vi "AcqDataQSMControlModule.vi"() -> ()   [LabVIEW 2013, in "main.lvlib"]
doc: "Læser 4 analoge differentierede datakanaler fra ADC'en og skriver dem til en TDMS-fil. Viser 2 af kanaler i grafer og 2 i søjler."
uses:
  main.lvlib
  Globals/DataAcqRecordPathGlobal.vi
  <vilib>/DAQmx/read.llb/DAQmx Read (Analog 1D DBL NChan 1Samp).vi
  Controls/Enum Globals.ctl
  Controls/Enum Variables.ctl
  Controls/Enum User Events.ctl
  <vilib>/DAQmx/create/channels.llb/DAQmx Create Channel (DO-Digital Output).vi
  <vilib>/DAQmx/write.llb/DAQmx Write (Digital 1D Bool NChan 1Samp 1Line).vi
panel:
  in  "Offset":dbl
  in  "Slide":dbl(slide) min=0.0 max=300.0 step=1.0 scale=0.3..300.0 scale format="%#_3g"
  out "Pressure":dbl(slide) scale=0.0..300.0 scale format="%#.3g"
  out "Red Chart":dbl(graph)
  out "Temperature":dbl caption="Temp"
  out "Blue Chart":dbl(graph)
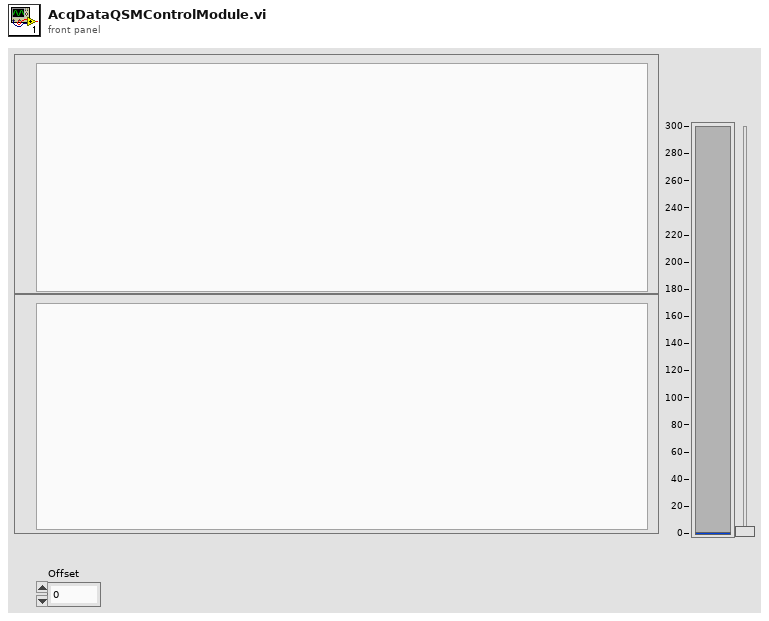
[diagram p1: front panel]
types:
  T1 = typedef "main.lvlib/Enum Globals.ctl" = enum16{"Init", "Set DataPath", "Set Freq", "Get"}
  T2 = typedef "main.lvlib/Enum User Events.ctl" = enum16{"User Event", "Init"}
  T3 = typedef "main.lvlib/Enum Variables.ctl" = enum16{"SetAcqFilter", "GetAcqFilter", "Set Filter", "Get Filter", "Set Height", "Get Height", "Set Blue Pressure", "Get Blue Pressure", "Set Red Pressure", "Get Red Pressure", "Init", "Reset Pressure", "Set Red Cursors", "Get Red Cursors", "Set Blue Cursors", "Get Blue Cursors", "Set Language", "Get Language", "Set Active Graphs", "Get ActiveGraphs", "Set Method", "Get Method", "Set Encryption", "Get Encryption", "Set ExcelVersion", "Get ExcelVersion", "Set DICOM Avail", "Get DICOM Avail", "Set DICOM Encode", "Get DICOM Encode", "Set JournalExport", "Get JournalExport", "Set Sequence", "Get Sequence", "Set DAQ Connected", "Get DAQ Connected", "Set Current Graph", "Get Current Graph", "Set General Settings", "Get Hyphenation", "Set Arm Calc Method", "Get Arm Calc Method", "Set Dicom Tags", "Get Dicom Tags", "Set BT Serial", "Get BT Serial", "Set BT Accepted Serials", "Get BT Accepted Serials", "Get BT License", "Set BT License"}
  T4 = cluster{"Freq Out":i32, "PressureCalibrationFactor":dbl, "RingOut":u16, "data":dbl[], "Value":dbl}
  T5 = cluster{"RingOut":u16, "PressureCalibrationFactor":dbl, "RingOut":u16, "data":dbl[], "Value":dbl}
  T6 = enum16{"open", "open or create", "create or replace", "create", "open (read-only)"}
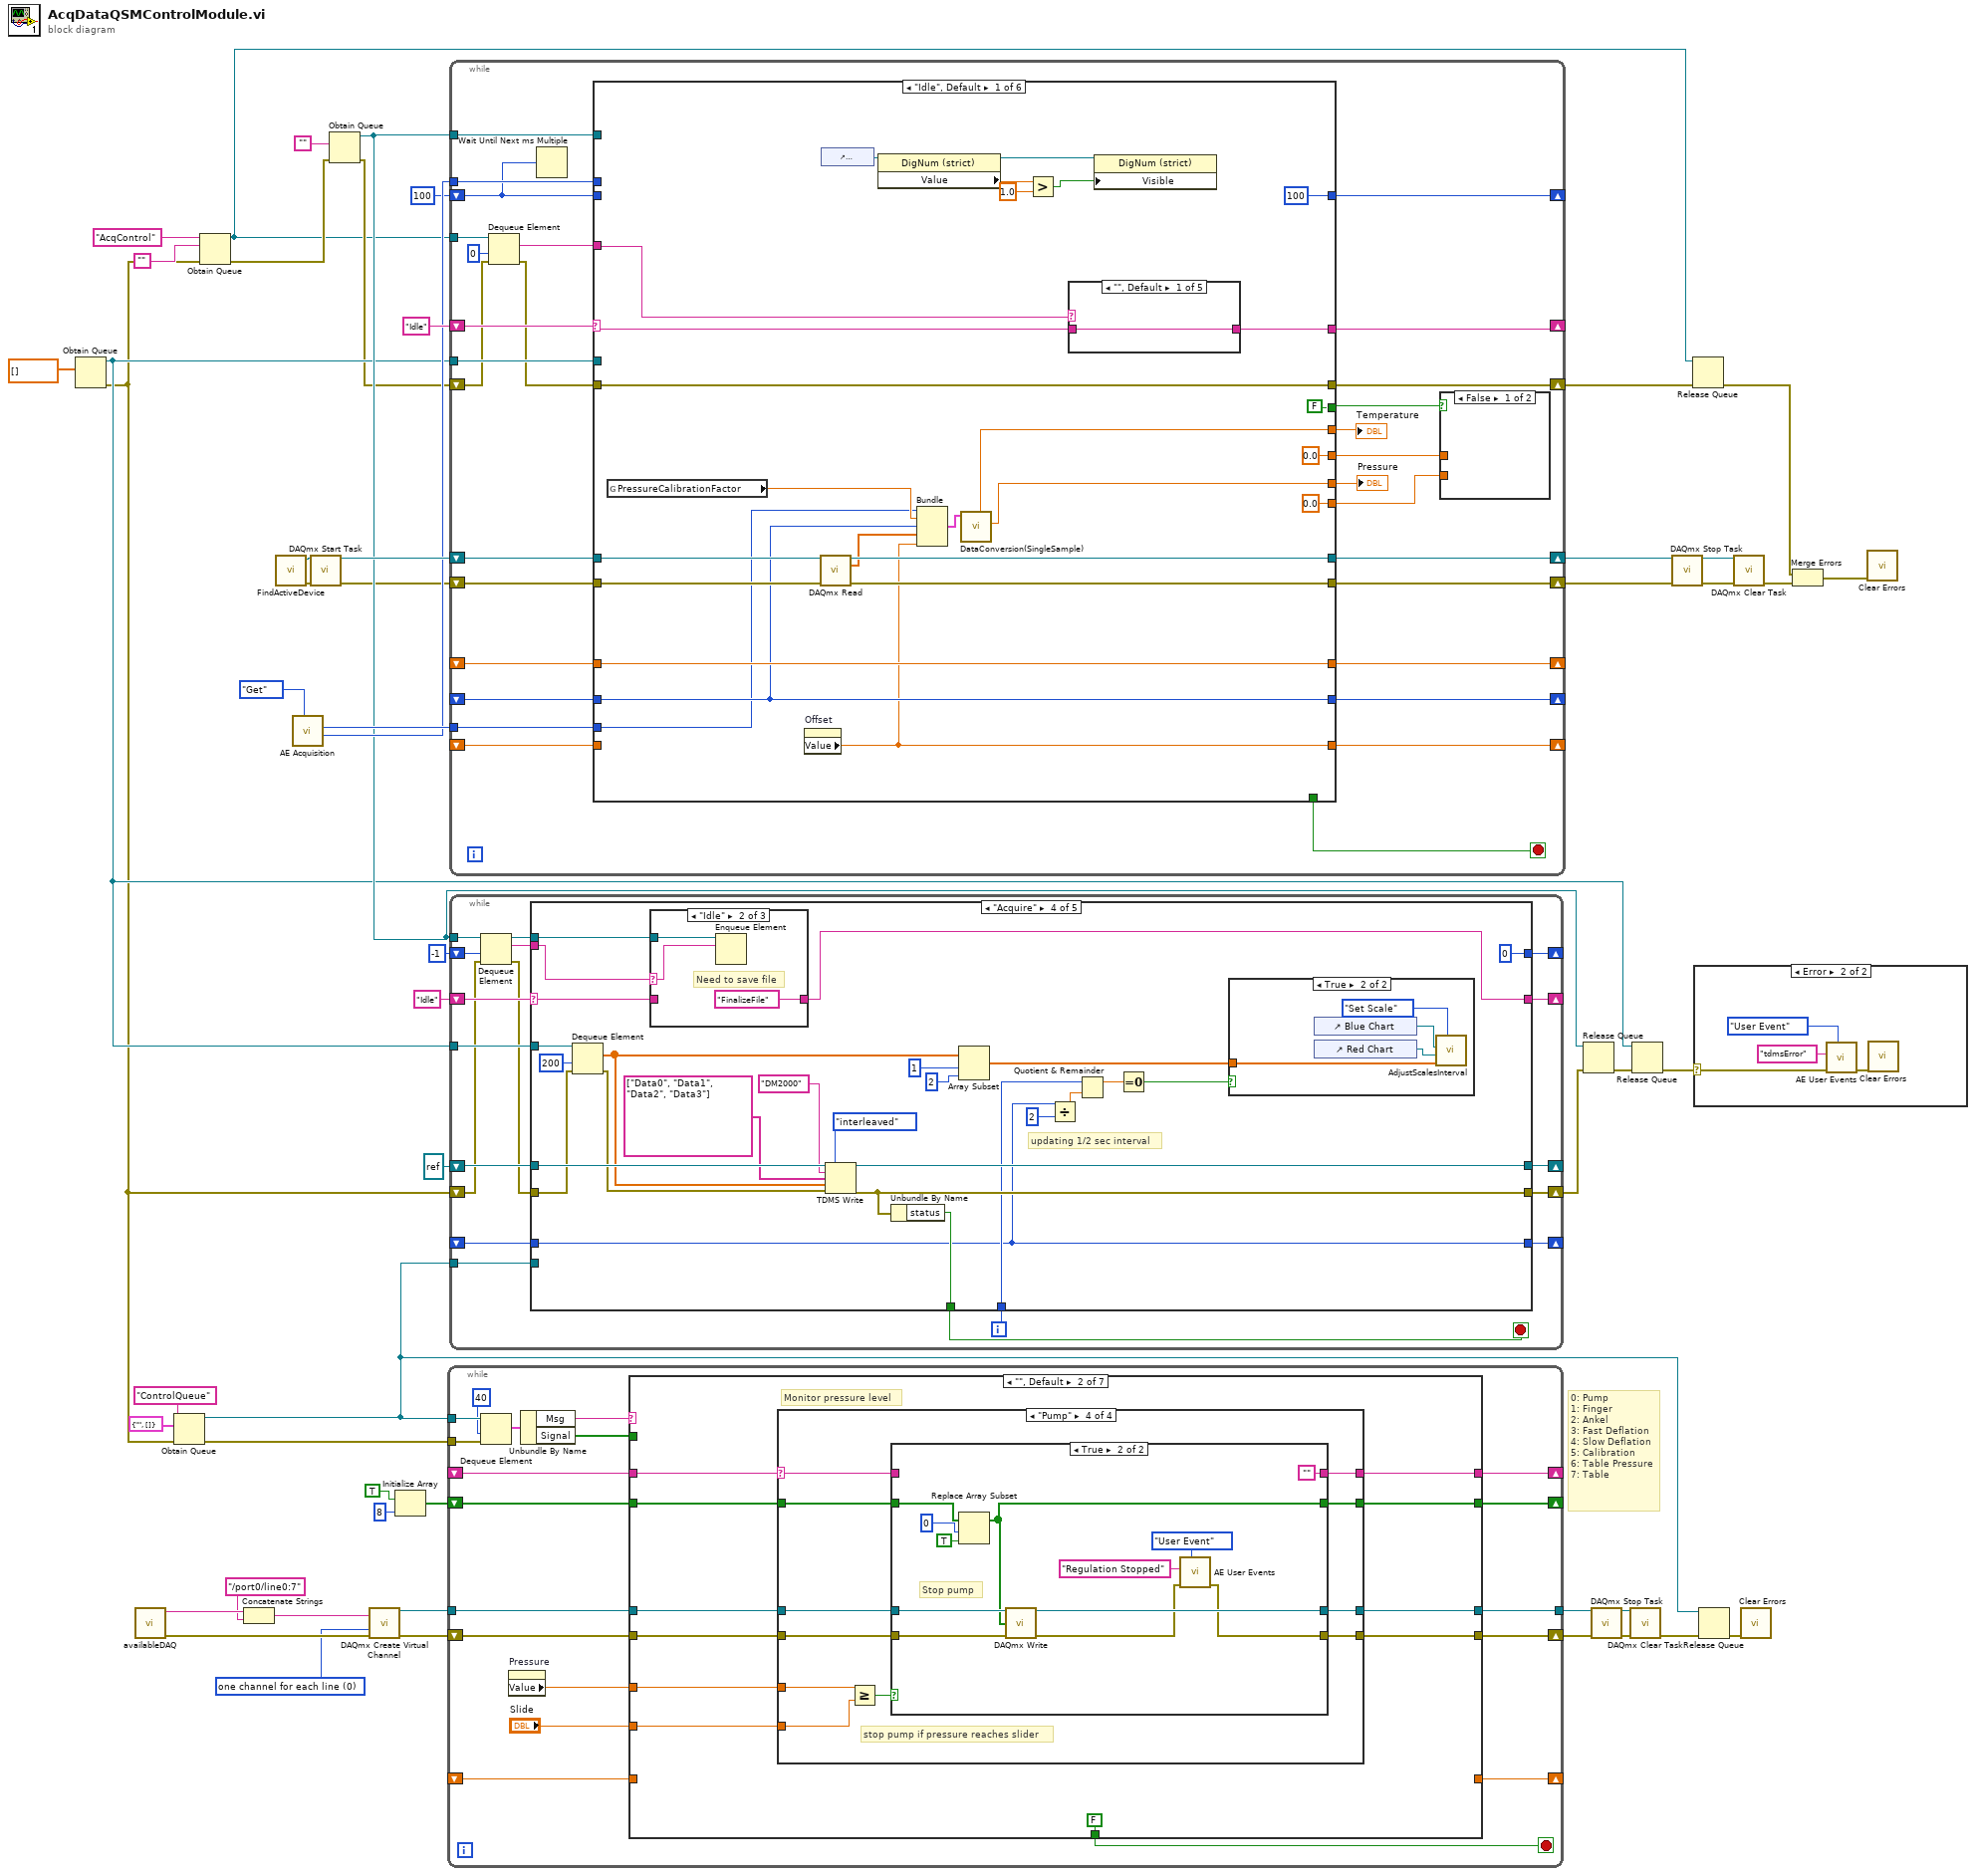
[diagram p0: block diagram]
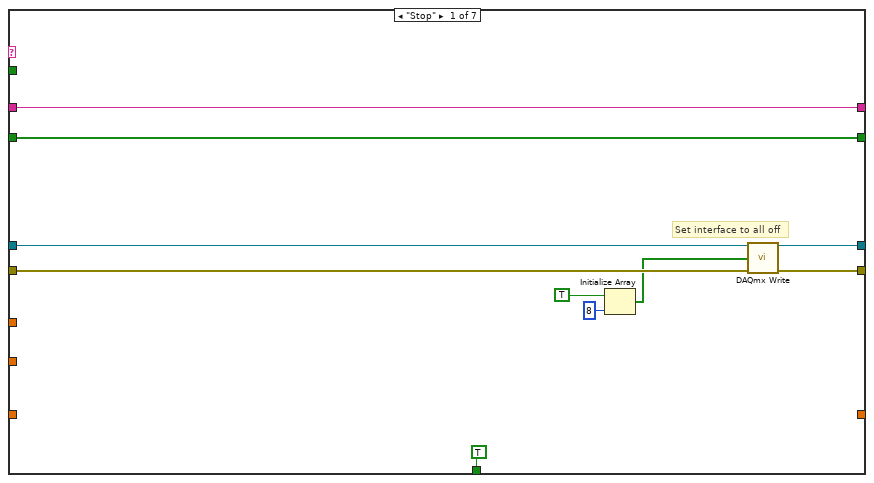
[diagram p2: hidden frame]
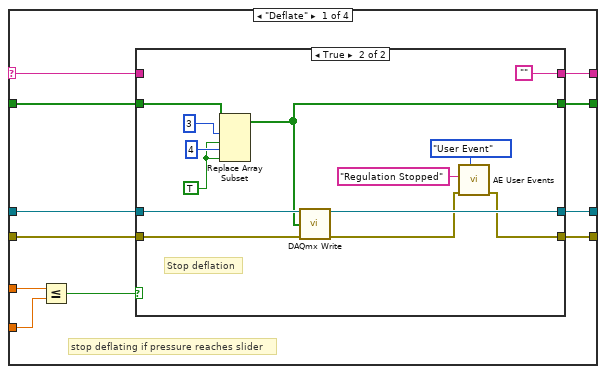
[diagram p3: hidden frame]
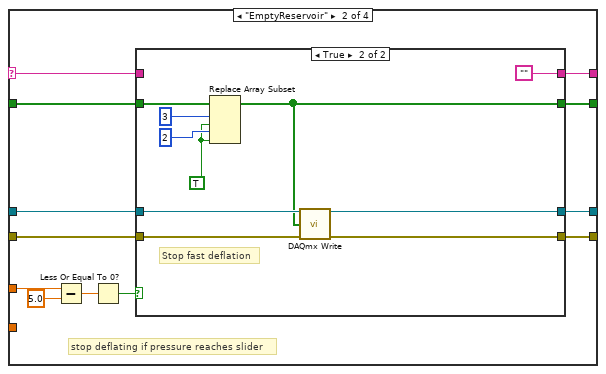
[diagram p5: hidden frame]
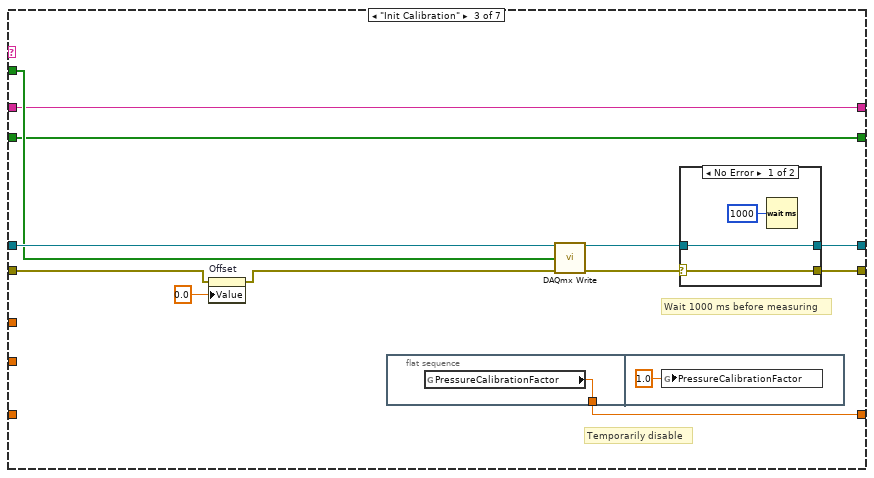
[diagram p9: hidden frame]
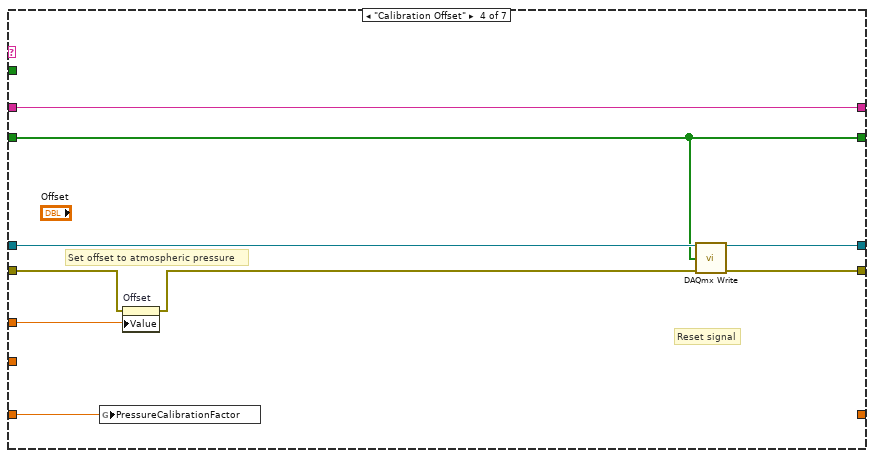
[diagram p11: hidden frame]
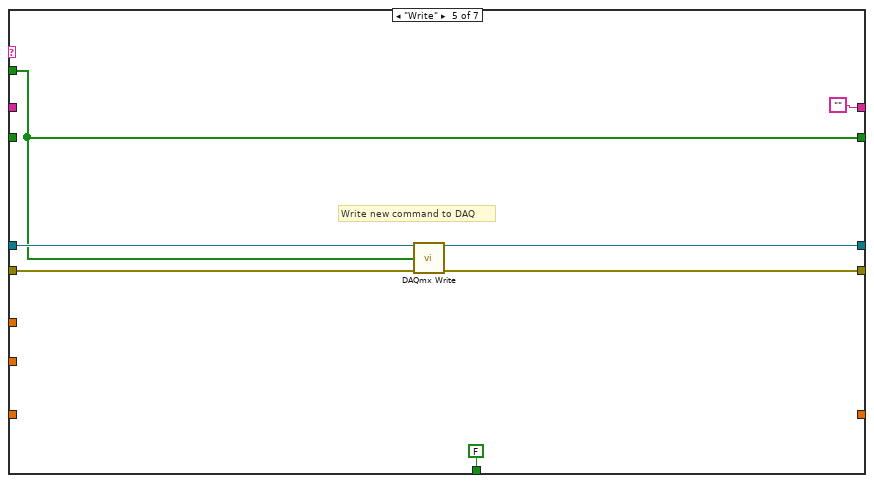
[diagram p12: hidden frame]
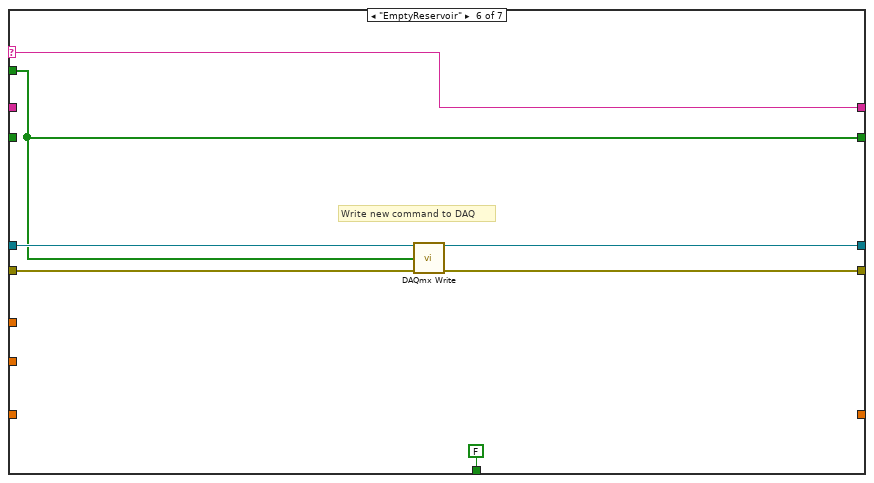
[diagram p13: hidden frame]
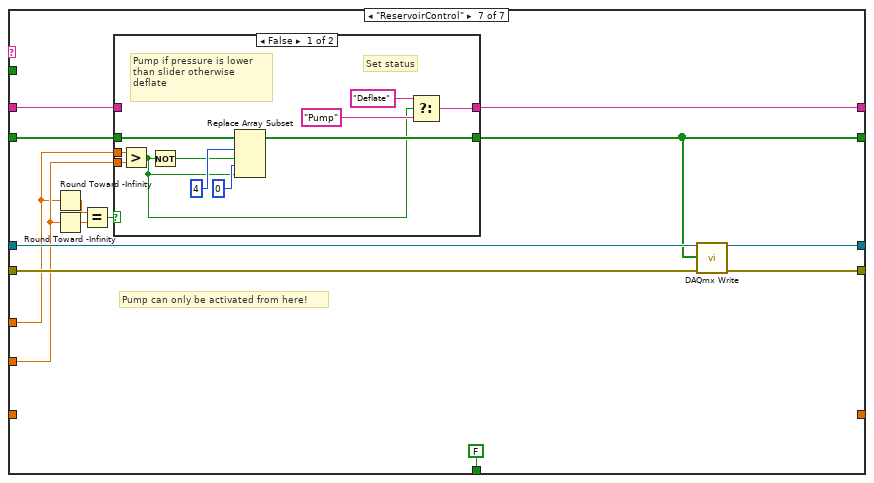
[diagram p14: hidden frame]
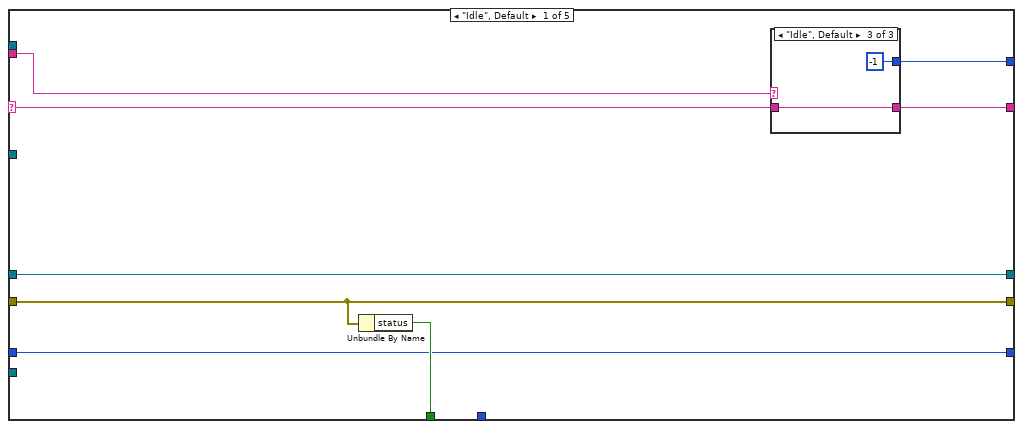
[diagram p17: hidden frame]
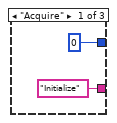
[diagram p18: hidden frame]
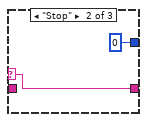
[diagram p19: hidden frame]
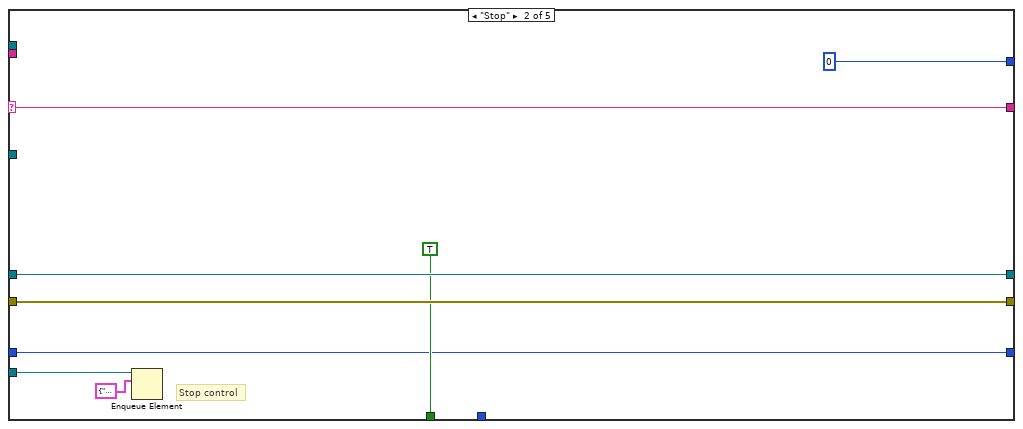
[diagram p20: hidden frame]
diagram:
  w8 = 0 items=["one channel for each line", "one channel for all lines"] ("line grouping")
  # "0: Pump\n1: Finger\n2: Ankel\n3: Fast Deflation\n4: Slow Deflation\n5: Calibration\n6: Table Pressure\n7: Table"
  n1 = Obtain Queue(element data type=dbl[] []) -> (queue out=w34:refnum<queue>, error out=w16:errorcluster)  [unwired: 4 in, 1 out]
  n2 = call "availableDAQ.vi"() -> ("error out"=w19:errorcluster, "DAQmx Device Name"=w21:tag)  [unwired: 10 in]
  n3 = Obtain Queue(name (unnamed)="ControlQueue", element data type=cluster{"Msg":string, "Signal":bool[]} {"Msg"="", "Signal"=[]}, error in (no error)=w16) -> (queue out=w4:refnum<queue>, error out=w7:errorcluster)  [unwired: 2 in, 1 out]
  n4 = Obtain Queue(name (unnamed)="AcqControl", element data type="", error in (no error)=w16) -> (queue out=w29:refnum<queue>, error out=w32:errorcluster)  [unwired: 2 in, 1 out]
  n5 = Concatenate Strings(w21, "/port0/line0:7" ("string")) -> (w18:string)
  n6 = call "FindActiveDevice.vi"() -> ("error out"=w37:errorcluster, "task out"=w38:refnum<k21>)  [unwired: 10 in]
  n7 = call "AE Acquisition.vi"("Action"=Enum_Globals."Get") -> ("Period(ms)"=w42:i32, "Freq Out"=w43:i32)  [unwired: 7 in, 2 out]
  n8 = call <vilib>:"DAQmx Start Task.vi"("task/channels in"=w38, "error in"=w37) -> ("task out"=w49:refnum<k21>, "error out"=w30:errorcluster)  [unwired: 12 in]
  n9 = Obtain Queue(element data type="", error in (no error)=w32) -> (queue out=w35:refnum<queue>, error out=w31:errorcluster)  [unwired: 3 in, 1 out]
  n10 = call-poly <vilib>:"DAQmx Create Virtual Channel.vi"("lines"=w18, "line grouping"=w8, "error in"=w19) -> ("task out"=w15:refnum<k21>, "error out"=w14:errorcluster)  [unwired: 11 in]
  n11 = Initialize Array(TRUE, 8 ("dimension size")) -> (w1:bool[])
  n12 = while {
    tunnel: w4 -> [w72]
    tunnel: w7 -> [w71]
    tunnel: w15 -> [w70]
    shift-right: [w68] -> w12
    shift-left: w14 -> [w69]
    tunnel: [w67] -> w13
    shift-right: [w62] -> _
    shift-left: w1 -> [w61]
    shift-right: [w57] -> _
    shift-left: _ -> [w60]
    shift-right: [w56] -> _
    shift-left: _ -> [w55]
    stop <- w64 stop-if-true
    n13 = Dequeue Element(queue=w72, timeout in ms (-1)=40, error in (no error)=w71) -> (element=w66:cluster{"Msg":string, "Signal":bool[]})  [unwired: 3 out]
    n14 = property on="Pressure" class="Slide (strict)"() -> ("Value"=w59:dbl)  [unwired: 2 in, 2 out]
    n15 = Unbundle By Name(w66) -> ("Msg"=w65:string, "Signal"=w54:bool[])
    n16 = case shown="\"\", Default" w65 {
      selector: w65 -> [_ _ _ _ _ w214 _]
      tunnel: w70 -> [w78 w92 w190 w203 w213 w220 w234]
      tunnel: w69 -> [w77 w91 w182 w200 w212 w219 w233]
      tunnel: [w79 w89 w185 w204 w210 w217 w231] -> w68
      tunnel: [w80 w90 w183 w205 w211 w218 w232] -> w67
      tunnel: [TRUE FALSE _ _ FALSE FALSE FALSE] -> w64
      tunnel: w54 -> [_ _ w189 _ w208 w215 _]
      tunnel: [w81 w87 w187 w202 w208 w215 w223] -> w62
      tunnel: w61 -> [w81 w88 w187 w202 _ _ w224]
      tunnel: w60 -> [w73 w86 w188 w206 _ _ w221]
      tunnel: w59 -> [_ w85 _ w201 _ _ w225]
      tunnel: "Slide" -> [_ w84 _ _ _ _ w227]
      tunnel: [w73 w83 w188 w206 "" w214 w222] -> w57
      tunnel: [_ _ w179 _ _ _ _] -> w56
      tunnel: w55 -> [_ _ _ w198 _ _ _]
      frame "Stop" {
        # "Set interface to all off"
        n17 = Initialize Array(TRUE, 8 ("dimension size")) -> (w74:bool[])
        n18 = call-poly <vilib>:"DAQmx Write.vi"("task/channels in"=w78, "data"=w74, "error in"=w77) -> ("task out"=w80:refnum<k21>, "error out"=w79:errorcluster)  [unwired: 10 in, 1 out]
      }
      frame "", Default {
        # "Monitor pressure level"
        n19 = case shown="\"Pump\"" w86 {
          selector: w86 -> [w95 w126 w151 w153]
          tunnel: w92 -> [w99 w128 w149 w162]
          tunnel: w91 -> [w100 w129 w148 w161]
          tunnel: [w102 w131 w149 w160] -> w90
          tunnel: [w101 w130 w148 w159] -> w89
          tunnel: w88 -> [w104 w133 w150 w157]
          tunnel: [w103 w132 w150 w156] -> w87
          tunnel: [w96 w127 w151 w152] -> w83
          tunnel: w85 -> [w97 w124 _ w155]
          tunnel: w84 -> [w98 _ _ w154]
          frame "Deflate" {
            # "stop deflating if pressure reaches slider"
            n20 = Less Or Equal?(x=w97, y=w98) -> (x <= y?=w94:bool)
            n21 = case shown="True" w94 {
              tunnel: w99 -> [w108 w121]
              tunnel: w100 -> [w107 w120]
              tunnel: [w108 w119] -> w102
              tunnel: [w107 w112] -> w101
              tunnel: w104 -> [w106 w118]
              tunnel: [w106 w109] -> w103
              tunnel: [w105 ""] -> w96
              tunnel: w95 -> [w105 _]
              frame False {
              }
              frame True {
                w110 = TRUE ("new element/subarray")
                # "Stop deflation"
                n22 = Replace Array Subset(array=w118, new element #1=w110, index #1=3 ("index"), new element #2=w110, index #2=4) -> (w109:bool[])
                n23 = call-poly <vilib>:"DAQmx Write.vi"("task/channels in"=w121, "data"=w109, "error in"=w120) -> ("task out"=w119:refnum<k21>, "error out"=w113:errorcluster)  [unwired: 10 in, 1 out]
                n24 = call "AE User Events.vi"("Action"=Enum_User_Events."User Event", "error in (no error)"=w113, "User Event"="Regulation Stopped") -> ("error out"=w112:errorcluster)  [unwired: 7 in, 1 out]
              }
            }
          }
          frame "EmptyReservoir" {
            # "stop deflating if pressure reaches slider"
            n25 = Subtract(x=w124, y=5.0) -> (x-y=w123:dbl)
            n26 = Less Or Equal To 0?(x=w123) -> (x <= 0?=w125:bool)
            n27 = case shown="True" w125 {
              tunnel: w128 -> [w137 w147]
              tunnel: w129 -> [w136 w146]
              tunnel: [w137 w145] -> w131
              tunnel: [w136 w141] -> w130
              tunnel: w133 -> [w135 w144]
              tunnel: [w135 w138] -> w132
              tunnel: [w134 ""] -> w127
              tunnel: w126 -> [w134 _]
              frame False {
              }
              frame True {
                w139 = TRUE ("new element/subarray")
                # "Stop fast deflation"
                n28 = Replace Array Subset(array=w144, new element #1=w139, index #1=3 ("index"), new element #2=w139, index #2=2 ("index")) -> (w138:bool[])
                n29 = call-poly <vilib>:"DAQmx Write.vi"("task/channels in"=w147, "data"=w138, "error in"=w146) -> ("task out"=w145:refnum<k21>, "error out"=w141:errorcluster)  [unwired: 10 in, 1 out]
              }
            }
          }
          frame "", Default {
          }
          frame "Pump" {
            # "stop pump if pressure reaches slider"
            n30 = Greater Or Equal?(x=w155, y=w154) -> (x >= y?=w158:bool)
            n31 = case shown="True" w158 {
              tunnel: w162 -> [w166 w178]
              tunnel: w161 -> [w165 w177]
              tunnel: [w166 w176] -> w160
              tunnel: [w165 w170] -> w159
              tunnel: w157 -> [w164 w173]
              tunnel: [w164 w167] -> w156
              tunnel: w153 -> [w163 _]
              tunnel: [w163 ""] -> w152
              frame False {
              }
              frame True {
                # "Stop pump"
                n32 = Replace Array Subset(array=w173, new element=TRUE ("new element/subarray"), index=0) -> (w167:bool[])
                n33 = call-poly <vilib>:"DAQmx Write.vi"("task/channels in"=w178, "data"=w167, "error in"=w177) -> ("task out"=w176:refnum<k21>, "error out"=w171:errorcluster)  [unwired: 10 in, 1 out]
                n34 = call "AE User Events.vi"("Action"=Enum_User_Events."User Event", "error in (no error)"=w171, "User Event"="Regulation Stopped") -> ("error out"=w170:errorcluster)  [unwired: 7 in, 1 out]
              }
            }
          }
        }
      }
      frame "Init Calibration" {
        # "Temporarily disable"
        # "Wait 1000 ms before measuring"
        n35 = property on="Offset" class="DigNum (strict)"(error in=w182, "Value"=0.0 ("Offset")) -> (error out=w181:errorcluster)  [unwired: 1 in, 1 out]
        n36 = flat-sequence {
          tunnel: [w191] -> w179
          frame #0 {
            n37 = global read "DataAcqRecordPathGlobal.vi" "PressureCalibrationFactor"() -> (w191:dbl)
          }
          frame #1 {
            n38 = global write "DataAcqRecordPathGlobal.vi" "PressureCalibrationFactor"(1.0 ("PressureCalibrationFactor")) -> ()
          }
        }
        n39 = call-poly <vilib>:"DAQmx Write.vi"("task/channels in"=w190, "data"=w189, "error in"=w181) -> ("task out"=w184:refnum<k21>, "error out"=w186:errorcluster)  [unwired: 10 in, 1 out]
        n40 = case shown="No Error" w186 {
          selector: w186 -> [w195 w197]
          tunnel: [w195 w197] -> w185
          tunnel: [w194 w196] -> w183
          tunnel: w184 -> [w194 w196]
          frame No Error {
            n41 = Wait (ms)(milliseconds to wait=u32 1000) -> ()  [unwired: 1 out]
          }
          frame Error {
          }
        }
      }
      frame "Calibration Offset" {
        # "Reset signal"
        # "Set offset to atmospheric pressure"
        n42 = global write "DataAcqRecordPathGlobal.vi" "PressureCalibrationFactor"(w198) -> ()
        n43 = property on="Offset" class="DigNum (strict)"(error in=w200, "Value"=w201) -> (error out=w199:errorcluster)  [unwired: 1 in, 1 out]
        n44 = call-poly <vilib>:"DAQmx Write.vi"("task/channels in"=w203, "data"=w202, "error in"=w199) -> ("task out"=w205:refnum<k21>, "error out"=w204:errorcluster)  [unwired: 10 in, 1 out]
      }
      frame "Write" {
        # "Write new command to DAQ"
        n45 = call-poly <vilib>:"DAQmx Write.vi"("task/channels in"=w213, "data"=w208, "error in"=w212) -> ("task out"=w211:refnum<k21>, "error out"=w210:errorcluster)  [unwired: 10 in, 1 out]
      }
      frame "EmptyReservoir" {
        # "Write new command to DAQ"
        n46 = call-poly <vilib>:"DAQmx Write.vi"("task/channels in"=w220, "data"=w215, "error in"=w219) -> ("task out"=w218:refnum<k21>, "error out"=w217:errorcluster)  [unwired: 10 in, 1 out]
      }
      frame "ReservoirControl" {
        # "Pump can only be activated from here!"
        n47 = Round Toward -Infinity(1:w225) -> (0:w226:dbl)
        n48 = Round Toward -Infinity(1:w227) -> (0:w228:dbl)
        n49 = Equal?(x=w226, y=w228) -> (x = y?=w229:bool)
        n50 = case shown="False" w229 {
          tunnel: w224 -> [w245 w247]
          tunnel: w225 -> [w243 _]
          tunnel: w227 -> [w242 _]
          tunnel: [w238 w247] -> w223
          tunnel: [w239 w246] -> w222
          tunnel: w221 -> [_ w246]
          frame False {
            # "Set status"
            # "Pump if pressure is lower than slider otherwise deflate"
            n51 = Greater?(x=w243, y=w242) -> (0:w236:bool)
            n52 = Not(x=w236) -> (.not. x?=w240:bool)
            n53 = Replace Array Subset(array=w245, new element #1=w240, index #1=4 ("index"), new element #2=w236, index #2=0 ("index")) -> (w238:bool[])
            n54 = Select(t="Deflate", s=w236, f="Pump") -> (s? t:f=w239:string)
          }
          frame True {
            # "Ignore if pressure = slide"
          }
        }
        n55 = call-poly <vilib>:"DAQmx Write.vi"("task/channels in"=w234, "data"=w223, "error in"=w233) -> ("task out"=w232:refnum<k21>, "error out"=w231:errorcluster)  [unwired: 10 in, 1 out]
      }
    }
  }
  n56 = while {
    shift-right: [w253] -> w50
    shift-left: w49 -> [w277]
    shift-right: [w252] -> w53
    shift-left: w30 -> [w276]
    shift-right: [w270] -> _
    shift-left: 100 ("Period(ms)") -> [w251]
    shift-right: [w255] -> w28
    shift-left: w31 -> [w257]
    shift-right: [w273] -> _
    shift-left: "Idle" -> [w274]
    tunnel: w43 -> [w269]
    tunnel: w42 -> [w268]
    shift-right: [w267] -> _
    shift-left: _ -> [w266]
    shift-right: [w262] -> _
    shift-left: _ -> [w261]
    tunnel: w29 -> [w260]
    tunnel: w35 -> [w258]
    tunnel: w34 -> [w275]
    shift-right: [w248] -> _
    shift-left: _ -> [w249]
    stop <- w254 stop-if-true
    n57 = Dequeue Element(queue=w260, timeout in ms (-1)=0, error in (no error)=w257) -> (element=w259:string, error out=w256:errorcluster)  [unwired: 2 out]
    n58 = Wait Until Next ms Multiple(millisecond multiple=w251) -> ()  [unwired: 1 out]
    n59 = case shown="\"Idle\", Default" w274 {
      selector: w274 -> [w298 _ w358 _ w410 w431]
      tunnel: [w305 w326 w366 w380 w416 w429] -> w252
      tunnel: w277 -> [w304 w329 w365 w383 w415 w430]
      tunnel: [w303 w330 w364 w384 w414 w430] -> w253
      tunnel: w276 -> [w302 w331 w363 w385 w413 w429]
      tunnel: [_ _ _ _ _ TRUE ("status")] -> w254
      tunnel: [100 w320 w357 w377 w404 w428] -> w270
      tunnel: w251 -> [_ _ w357 _ w404 w428]
      tunnel: w275 -> [_ _ w361 _ _ _]
      tunnel: [w301 w317 w348 w396 w409 w421] -> w255
      tunnel: w256 -> [w301 w317 w362 w396 w409 w421]
      tunnel: [w286 0.0 w353 0.0 w406 _] -> w272
      tunnel: [w300 0.0 ("Temperature") w360 0.0 ("Temperature") w412 _] -> w271
      tunnel: [w297 "Acquire" w359 "Test" w411 w431] -> w273
      tunnel: [0.0 ("Blue Data") _ w355 _ w407 _] -> w263
      tunnel: [0.0 ("Red Data") _ w354 _ w408 _] -> w264
      tunnel: [FALSE FALSE TRUE FALSE TRUE FALSE] -> w265
      tunnel: w269 -> [w281 w324 w344 w375 w399 _]
      tunnel: w268 -> [_ w320 _ w377 _ _]
      tunnel: [w288 w314 w345 w374 w398 w425] -> w267
      tunnel: w266 -> [w288 _ w345 _ w398 w425]
      tunnel: [w283 w313 w346 w372 w397 w424] -> w262
      tunnel: w261 -> [w283 w315 w346 _ w397 w424]
      tunnel: w259 -> [w287 _ w350 _ w403 _]
      tunnel: w258 -> [_ w319 w349 _ _ w423]
      tunnel: w249 -> [_ w311 w342 w371 w400 w420]
      tunnel: [w280 w311 w342 w371 w400 w420] -> w248
      frame "Idle", Default {
        n60 = global read "DataAcqRecordPathGlobal.vi" "PressureCalibrationFactor"() -> (w282:dbl)
        n61 = property on="Offset" class="DigNum (strict)"() -> ("Value"=w280:dbl)  [unwired: 2 in, 2 out]
        n62 = call-poly <vilib>:"DAQmx Read.vi"("task/channels in"=w304, "error in"=w302) -> ("task out"=w303:refnum<k21>, "data"=w284:dbl[], "error out"=w305:errorcluster)  [unwired: 11 in]
        n63 = control-ref of="Temperature"() -> (w293:refnum<vi>)
        n64 = property class="DigNum (strict)"(reference=w293) -> (reference out=w292:refnum<vi>, "Value"=w291:dbl)  [unwired: 1 in, 1 out]
        n65 = Bundle("Freq Out"=w281, "PressureCalibrationFactor"=w282, "RingOut"=w283, "data"=w284, "Value"=w280) -> (w285:T4)  [unwired: 1 in]
        n66 = call "DataConversion(SingleSample).vi"("input cluster"=w285) -> ("Temperature"=w300:dbl, "Pressure"=w286:dbl)  [unwired: 5 in, 3 out]
        n67 = Greater?(x=w291, y=1.0) -> (0:w289:bool)
        n68 = case shown="\"\", Default" w287 {
          tunnel: w298 -> [w306 w307 _ _ _]
          tunnel: [w306 w307 "Initialize" "Stop" "InitTest"] -> w297
          frame "", Default {
          }
          frame "Idle" {
          }
          frame "Acquire" {
          }
          frame "Stop" {
          }
          frame "Test" {
          }
        }
        n69 = property class="DigNum (strict)"(reference=w292, "Visible"=w289) -> ()  [unwired: 1 in, 2 out]
      }
      frame "Initialize" {
        w337 = dbl[] [] ("Value")
        n70 = global read "DataAcqRecordPathGlobal.vi" "PressureCalibrationFactor"() -> (w314:dbl)
        n71 = Enqueue Element(queue=w319, element="Acquire") -> ()  [unwired: 2 in, 3 out]
        n72 = Reciprocal(x=w324) -> (1/x=w336:dbl)
        n73 = control-ref of="Red Chart"() -> (w328:refnum<vi>)
        n74 = control-ref of="Blue Chart"() -> (w327:refnum<vi>)
        n75 = call "AE Variables.vi"("Action"=Enum_Variables."Get ActiveGraphs") -> ("RingOut"=w313:u16)  [unwired: 11 in, 7 out]
        n76 = call-poly <vilib>:"DAQmx Read.vi"("task/channels in"=w329, "error in"=w331) -> ("task out"=w330:refnum<k21>, "data"=w312:dbl[], "error out"=w326:errorcluster)  [unwired: 11 in]
        n77 = property class="WFChart (strict)"(reference=w328, "History Data"=w337, "XScale.Multiplier"=w336) -> (reference out=w323:refnum<vi>)  [unwired: 1 in, 1 out]
        n78 = property class="WFChart (strict)"(reference=w327, "History Data"=w337, "XScale.Multiplier"=w336) -> (reference out=w322:refnum<vi>)  [unwired: 1 in, 1 out]
        n79 = Bundle("RingOut"=w315, "PressureCalibrationFactor"=w314, "RingOut"=w313, "data"=w312, "Value"=w311) -> (w316:T5)  [unwired: 1 in]
        n80 = call "DataConversion(SingleSample).vi"("input cluster"=w316, "Init"=TRUE) -> ("Red Data"=w333:dbl, "Blue Data"=w334:dbl)  [unwired: 4 in, 3 out]
        n81 = Build Array(w334, w333) -> (w332:dbl[])
        n82 = call "AdjustScalesInterval.vi"("Action"=enum16{"Init", "Set Scale"}."Init", "Data"=w332, "WFChart Refnum 2"=w323, "WFChart Refnum"=w322) -> ()  [unwired: 8 in]
      }
      frame "Acquire" {
        n83 = call-poly <vilib>:"DAQmx Read.vi"("task/channels in"=w365, "error in"=w363) -> ("task out"=w364:refnum<k21>, "data"=w347:dbl[], "error out"=w366:errorcluster)  [unwired: 11 in]
        n84 = Bundle("Freq Out"=w344, "PressureCalibrationFactor"=w345, "RingOut"=w346, "data"=w347, "Value"=w342) -> (w343:T4)  [unwired: 1 in]
        n85 = call "DataConversion(SingleSample).vi"("input cluster"=w343, "Init"=FALSE) -> ("Temperature"=w360:dbl, "All Data"=w356:dbl[], "Red Data"=w354:dbl, "Pressure"=w353:dbl, "Blue Data"=w355:dbl)  [unwired: 4 in]
        n86 = Enqueue Element(queue=w361, element=w356, error in (no error)=w362) -> (error out=w348:errorcluster)  [unwired: 1 in, 2 out]
        n87 = case shown="\"\", Default" w350 {
          selector: w350 -> [_ w368 w370]
          tunnel: [w367 w368 w370] -> w359
          tunnel: w358 -> [w367 _ _]
          tunnel: w349 -> [_ w369 _]
          frame "", Default {
          }
          frame "Idle" {
            n88 = Enqueue Element(queue=w369, element=w368) -> ()  [unwired: 2 in, 3 out]
          }
          frame "Stop" {
          }
        }
      }
      frame "InitTest" {
        w391 = dbl[] [] ("Value")
        n89 = Reciprocal(x=w375) -> (1/x=w390:dbl)
        n90 = global read "DataAcqRecordPathGlobal.vi" "PressureCalibrationFactor"() -> (w374:dbl)
        n91 = call "AE Variables.vi"("Action"=Enum_Variables."Get ActiveGraphs") -> ("RingOut"=w372:u16)  [unwired: 11 in, 7 out]
        n92 = control-ref of="Red Chart"() -> (w382:refnum<vi>)
        n93 = control-ref of="Blue Chart"() -> (w381:refnum<vi>)
        n94 = call-poly <vilib>:"DAQmx Read.vi"("task/channels in"=w383, "error in"=w385) -> ("task out"=w384:refnum<k21>, "data"=w373:dbl[], "error out"=w380:errorcluster)  [unwired: 11 in]
        n95 = Bundle("Freq Out"=w375, "PressureCalibrationFactor"=w374, "RingOut"=w372, "data"=w373, "Value"=w371) -> (w376:T4)  [unwired: 1 in]
        n96 = call "DataConversion(SingleSample).vi"("input cluster"=w376, "Init"=TRUE) -> ("Red Data"=w387:dbl, "Blue Data"=w388:dbl)  [unwired: 4 in, 3 out]
        n97 = Build Array(w388, w387) -> (w386:dbl[])
        n98 = property class="WFChart (strict)"(reference=w382, "History Data"=w391, "XScale.Multiplier"=w390) -> ()  [unwired: 1 in, 2 out]
        n99 = property class="WFChart (strict)"(reference=w381, "History Data"=w391, "XScale.Multiplier"=w390) -> ()  [unwired: 1 in, 2 out]
        n100 = call "AdjustScalesInterval.vi"("Action"=enum16{"Init", "Set Scale"}."Init", "Data"=w386, "WFChart Refnum 2"=w382, "WFChart Refnum"=w381) -> ()  [unwired: 8 in]
      }
      frame "Test" {
        n101 = call-poly <vilib>:"DAQmx Read.vi"("task/channels in"=w415, "error in"=w413) -> ("task out"=w414:refnum<k21>, "data"=w401:dbl[], "error out"=w416:errorcluster)  [unwired: 11 in]
        n102 = Bundle("Freq Out"=w399, "PressureCalibrationFactor"=w398, "RingOut"=w397, "data"=w401, "Value"=w400) -> (w402:T4)  [unwired: 1 in]
        n103 = call "DataConversion(SingleSample).vi"("input cluster"=w402) -> ("Temperature"=w412:dbl, "Red Data"=w408:dbl, "Pressure"=w406:dbl, "Blue Data"=w407:dbl)  [unwired: 5 in, 1 out]
        n104 = case shown="\"False\", Default" w403 {
          tunnel: [w417 "Idle" "Stop"] -> w411
          tunnel: w410 -> [w417 _ _]
          frame "False", Default {
          }
          frame "Idle" {
          }
          frame "Stop" {
          }
        }
      }
      frame "Stop" {
        n105 = Enqueue Element(queue=w423, element="Stop") -> ()  [unwired: 2 in, 3 out]
      }
    }
    "Pressure" <- w272
    "Temperature" <- w271
    n106 = case shown="False" w265 {
      tunnel: w264 -> [_ w279]
      tunnel: w263 -> [_ w278]
      frame False {
      }
      frame True {
        "Blue Chart" <- w278
        "Red Chart" <- w279
      }
    }
  }
  n107 = while {
    tunnel: w34 -> [w449]
    shift-right: [w447] -> _
    shift-left: refnum<k34> refnum ("tdms file out") -> [w448]
    shift-right: [w446] -> w45
    shift-left: w16 -> [w435]
    shift-right: [w443] -> _
    shift-left: "Idle" -> [w444]
    shift-right: [w441] -> _
    shift-left: _ -> [w440]
    tunnel: w35 -> [w439]
    shift-right: [w436] -> _
    shift-left: -1 -> [w437]
    tunnel: w4 -> [w432]
    i -> [w442]
    stop <- w445 stop-if-true
    n108 = Dequeue Element(queue=w439, timeout in ms (-1)=w437, error in (no error)=w435) -> (queue out=w433:refnum<queue>, element=w438:string, error out=w434:errorcluster)  [unwired: 1 out]
    n109 = case shown="\"Acquire\"" w444 {
      selector: w444 -> [w455 w471 _ w502 _]
      tunnel: w449 -> [_ _ _ w503 w521]
      tunnel: w448 -> [w457 w470 _ w506 w525]
      tunnel: [w457 w470 w476 w507 w525] -> w447
      tunnel: [w454 w469 w477 w505 w526] -> w446
      tunnel: w434 -> [w454 w469 w479 w499 w520]
      tunnel: [w453 TRUE ("status") w478 w504 w527] -> w445
      tunnel: [w456 w471 "Acquire" w496 w522] -> w443
      tunnel: w442 -> [_ _ _ w491 _]
      tunnel: [w452 w467 w473 w486 w524] -> w441
      tunnel: w440 -> [w452 w467 _ w486 w524]
      tunnel: w438 -> [w451 _ _ w484 w522]
      tunnel: [w450 0 0 0 100] -> w436
      tunnel: w433 -> [_ _ _ w483 _]
      tunnel: w432 -> [_ w465 _ _ _]
      frame "Idle", Default {
        n110 = Unbundle By Name(w454) -> ("status"=w453:bool)
        n111 = case shown="\"Idle\", Default" w451 {
          selector: w451 -> [_ w460 _]
          tunnel: ["Initialize" w460 w463] -> w456
          tunnel: w455 -> [_ _ w463]
          tunnel: [0 0 -1] -> w450
          frame "Acquire" {
          }
          frame "Stop" {
          }
          frame "Idle", Default {
          }
        }
      }
      frame "Stop" {
        # "Stop control"
        n112 = Enqueue Element(queue=w465, element=cluster{"Msg":string, "Signal":bool[]} {"Msg"="Stop", "Signal"=[]}) -> ()  [unwired: 2 in, 3 out]
      }
      frame "Initialize" {
        n113 = global read "DataAcqRecordPathGlobal.vi" "DataAcqRecordPath"() -> (w481:path)
        n114 = TDMS Open(8:w479, 10:T6."create or replace" ("operation (0:open)"), 11:w481) -> (0:w477:errorcluster, 3:w476:refnum<k34>)  [unwired: 4 in]
        n115 = Unbundle By Name(w477) -> ("status"=w478:bool)
        n116 = call "AE Acquisition.vi"("Action"=Enum_Globals."Get") -> ("Freq Out"=w473:i32)  [unwired: 7 in, 3 out]
      }
      frame "Acquire" {
        # "updating 1/2 sec interval"
        n117 = Dequeue Element(queue=w503, timeout in ms (-1)=200, error in (no error)=w499) -> (element=w490:dbl[], error out=w498:errorcluster)  [unwired: 2 out]
        n118 = case shown="\"Idle\"" w484 {
          selector: w484 -> [_ w513 w516]
          tunnel: [w512 "FinalizeFile" "FinalizeFile"] -> w496
          tunnel: w502 -> [w512 _ _]
          tunnel: w483 -> [_ w514 w517]
          frame "", Default {
          }
          frame "Idle" {
            # "Need to save file"
            n119 = Enqueue Element(queue=w514, element=w513) -> ()  [unwired: 2 in, 3 out]
          }
          frame "Stop" {
            # "Need to save file"
            n120 = Enqueue Element(queue=w517, element=w516) -> ()  [unwired: 2 in, 3 out]
          }
        }
        n121 = TDMS Write(0:w506, 1:enum16{"decimated", "interleaved"}."interleaved" ("data layout (0:decimated)"), 5:"DM2000", 7:string[] ["Data0", "Data1", "Data2", "Data3"], 9:w490, 11:w498) -> (4:w507:refnum<k34>, 15:w505:errorcluster)  [unwired: 2 out]
        n122 = Unbundle By Name(w505) -> ("status"=w504:bool)
        n123 = Array Subset(array=w490, index=1, length=2) -> (w487:dbl[])
        n124 = Divide(x=w486, y=2) -> (x/y=w494:dbl)
        n125 = Quotient & Remainder(x=w491, y=w494) -> (x-y*floor(x/y)=w493:dbl)  [unwired: 1 out]
        n126 = Equal To 0?(x=w493) -> (x = 0?=w492:bool)
        n127 = case shown="True" w492 {
          tunnel: w487 -> [_ w511]
          frame False {
          }
          frame True {
            n128 = control-ref of="Blue Chart"() -> (w509:refnum<vi>)
            n129 = control-ref of="Red Chart"() -> (w510:refnum<vi>)
            n130 = call "AdjustScalesInterval.vi"("Action"=enum16{"Init", "Set Scale"}."Set Scale", "Data"=w511, "WFChart Refnum 2"=w510, "WFChart Refnum"=w509) -> ()  [unwired: 8 in]
          }
        }
      }
      frame "FinalizeFile" {
        n131 = Flush Queue(queue=w521, error in (no error)=w520) -> (error out=w519:errorcluster)  [unwired: 2 out]
        n132 = TDMS Close(8:w519, 11:w525) -> (0:w526:errorcluster)  [unwired: 1 out]
        n133 = Unbundle By Name(w526) -> ("status"=w527:bool)
      }
    }
  }
  n134 = Release Queue(queue=w35, error in (no error)=w45) -> (error out=w33:errorcluster)  [unwired: 1 in, 2 out]
  n135 = call <vilib>:"DAQmx Stop Task.vi"("task/channels in"=w13, "error in"=w12) -> ("task out"=w11:refnum<k21>, "error out"=w10:errorcluster)  [unwired: 12 in]
  n136 = call <vilib>:"DAQmx Clear Task.vi"("task in"=w11, "error in"=w10) -> ("error out"=w6:errorcluster)  [unwired: 13 in]
  n137 = Release Queue(queue=w34, error in (no error)=w33) -> (error out=w26:errorcluster)  [unwired: 1 in, 2 out]
  n138 = call <vilib>:"DAQmx Stop Task.vi"("task/channels in"=w50, "error in"=w53) -> ("task out"=w52:refnum<k21>, "error out"=w51:errorcluster)  [unwired: 12 in]
  n139 = Release Queue(queue=w29, error in (no error)=w28) -> (error out=w24:errorcluster)  [unwired: 1 in, 2 out]
  n140 = case shown="Error" w26 {
    selector: w26 -> [_ w529]
    frame No Error {
    }
    frame Error {
      n141 = call "AE User Events.vi"("Action"=Enum_User_Events."User Event", "error in (no error)"=w529, "User Event"="tdmsError") -> ("error out"=w528:errorcluster)  [unwired: 7 in, 1 out]
      n142 = call <vilib>:"Clear Errors.vi"("error in (no error)"=w528) -> ()  [unwired: 6 in, 1 out]
    }
  }
  n143 = Release Queue(queue=w4, error in (no error)=w6) -> (error out=w5:errorcluster)  [unwired: 1 in, 2 out]
  n144 = call <vilib>:"DAQmx Clear Task.vi"("task in"=w52, "error in"=w51) -> ("error out"=w25:errorcluster)  [unwired: 13 in]
  n145 = call <vilib>:"Clear Errors.vi"("error in (no error)"=w5) -> ()  [unwired: 6 in, 1 out]
  n146 = Merge Errors(w24, w25) -> (w23:errorcluster)
  n147 = call <vilib>:"Clear Errors.vi"("error in (no error)"=w23) -> ()  [unwired: 6 in, 1 out]
